vi "SORT 2D ARRAY.vi"() -> ()   [LabVIEW 2018]
uses:
  ce05e502-6c63-4215-b423-1d24f1764da2.vi
  <vilib>/Array/Sort 2D Array - Pop Stack.vi
  <vilib>/Array/Sort 2D Array - Push Stack.vi
panel:
  out "sorted array":dbl[](array[numeric])
  out "appended array":dbl[][](array[numeric])
  in  "Array 2":dbl[][](array[numeric])
  out "sorted 2D array":dbl[][](array[numeric])
  in  "Array":dbl[][](array[numeric])
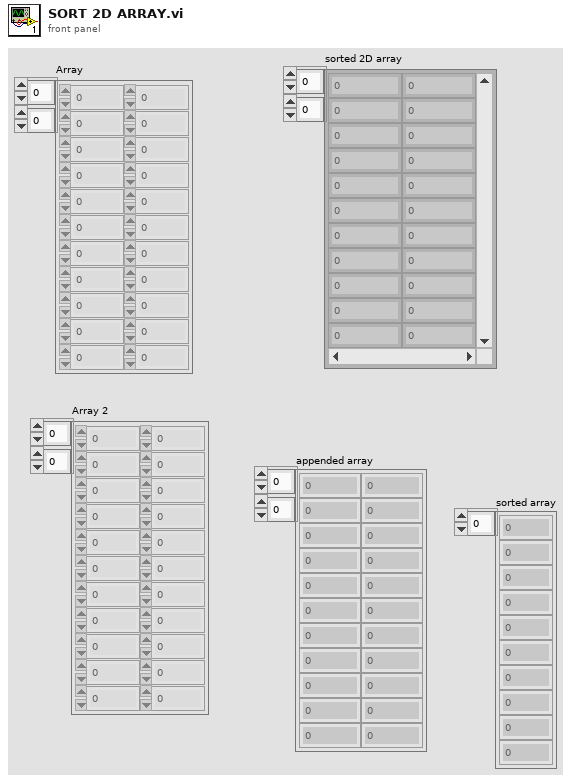
[diagram p1: front panel]
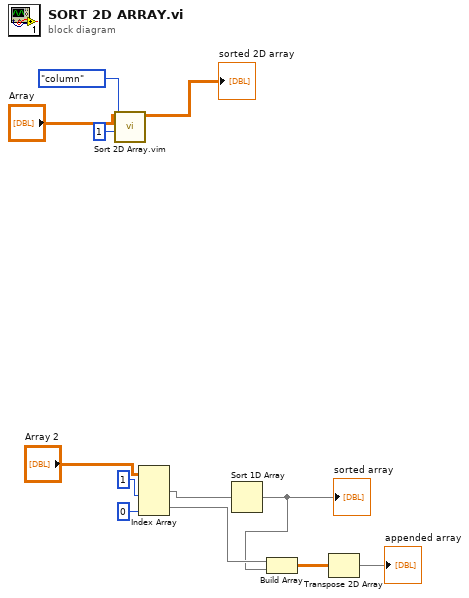
[diagram p0: block diagram]
diagram:
  n1 = call "Sort 2D Array.vim"("index"=1, "dimension to index (column)"=enum16{"column", "row"}."column", "2D array"="Array") -> ("sorted 2D array"=→"sorted 2D array":dbl[][])  [unwired: 7 in, 1 out]
  n2 = Index Array(array="Array 2", index (col) #1=1 ("disabled index (col)"), index (col) #2=0 ("index (col)")) -> (element #1=w6:dbl[], element #2=w5:dbl[])  [unwired: 2 in]
  n3 = Sort 1D Array(array=w6) -> (sorted array=w2:dbl[])
  "sorted array" <- w2
  n4 = Build Array(w5, w2) -> (w4:dbl[][])
  n5 = Transpose 2D Array(2D array=w4) -> (transposed array=→"appended array":dbl[][])
